vi "Sprite.vi"(5 "Pause":bool, 7 "Skip":bool, 8 "error in (no error)":errorcluster, 9 "Skip to Frame":i32=1 min=1, 10 "Sprite Sequence":T1, 11 "Sprite Name":string) -> (0 "error out":errorcluster, 1 "Next Fame":i32, 2 "Frame Output":picture, 3 "Sprite Name Out":string)   [LabVIEW 2020]
uses:
  Stickman State.ctl
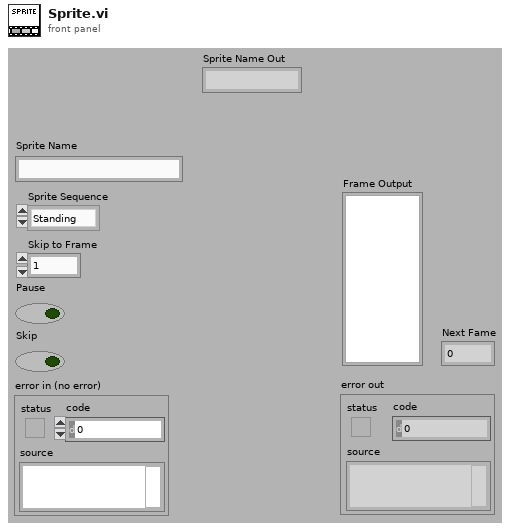
[diagram p1: front panel]
types:
  T1 = typedef "Stickman State.ctl" = enum16{"Standing", "Walking"}
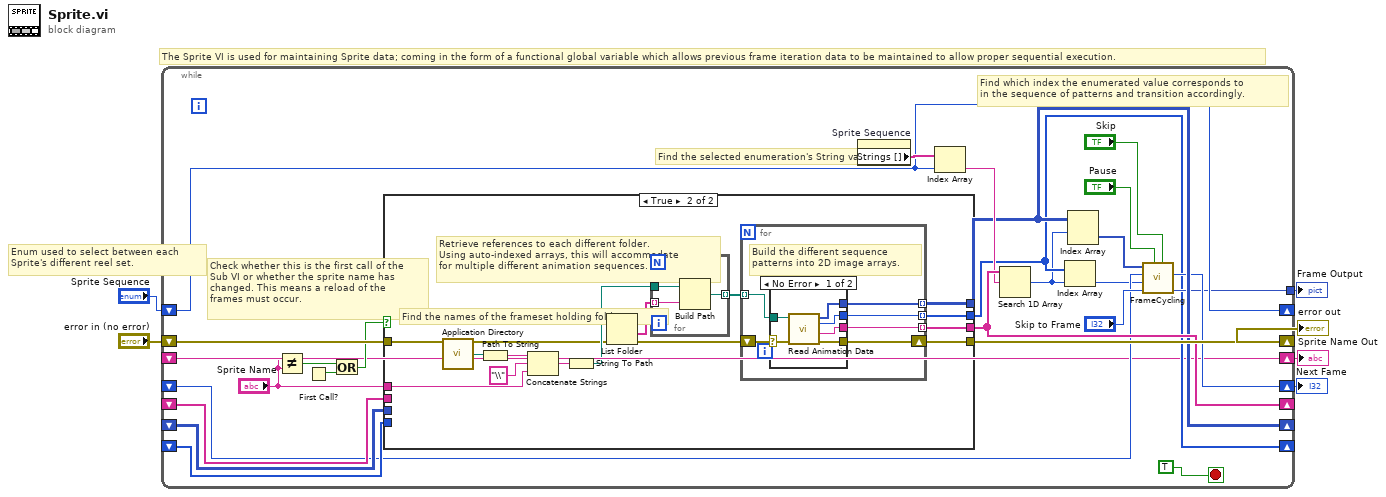
[diagram p0: block diagram]
diagram:
  # "Enum used to select between each\nSprite's different reel set."
  # "The Sprite VI is used for maintaining Sprite data; coming in the form of a functional global variable which allows previous frame iteration data to be maintained to allow proper sequential execution."
  n1 = while {
    shift-right: [w17] -> w2
    shift-left: _ -> [w18]
    shift-right: [w26] -> _
    shift-left: "Sprite Sequence" -> [w26]
    shift-right: [w23] -> _
    shift-left: _ -> [w31]
    shift-right: [w30] -> w4
    shift-left: "error in (no error)" -> [w32]
    shift-right: [w14] -> _
    shift-left: _ -> [w29]
    shift-right: [w25] -> _
    shift-left: _ -> [w28]
    tunnel: [w16] -> w3
    shift-right: ["Sprite Name"] -> w1
    shift-left: _ -> [w8]
    stop <- TRUE stop-if-true
    # "Find which index the enumerated value corresponds to\nin the sequence of patterns and transition accordingly."
    # "Find the selected enumeration's String value."
    # "Check whether this is the first call of the\nSub VI or whether the sprite name has\nchanged. This means a reload of the\nframes must occur."
    n2 = Not Equal?(x=w8, y="Sprite Name") -> (x != y?=w11:bool)
    n3 = First Call?() -> (First Call?: T/F=w10:bool)
    n4 = Or(x=w11, y=w10) -> (x .or. y?=w9:bool)
    n5 = case shown="True" w9 {
      tunnel: [w35 w50] -> w23
      tunnel: w32 -> [w36 w41]
      tunnel: w31 -> [w35 _]
      tunnel: [w36 w49] -> w30
      tunnel: [w34 w48] -> w14
      tunnel: [w33 w47] -> w25
      tunnel: w29 -> [w34 _]
      tunnel: w28 -> [w33 _]
      tunnel: "Sprite Name" -> [_ w38]
      frame False {
      }
      frame True {
        # "Retrieve references to each different folder.\nUsing auto-indexed arrays, this will accommodate\nfor multiple different animation sequences."
        # "Find the names of the frameset holding folders."
        n6 = call <vilib>:"Application Directory.vi"() -> ("Application Directory"=w37:path)
        n7 = Path To String(path=w37) -> (string=w46:string)
        n8 = Concatenate Strings(w46, "\\" ("string"), w38) -> (w45:string)
        n9 = String To Path(string=w45) -> (path=w43:path)
        n10 = List Folder(path=w43, error in=w41) -> (folder names=w44:string[], error out=w40:errorcluster)  [unwired: 2 in, 2 out]
        n11 = for {
          tunnel: w44 -> [w52] mode=indexing
          tunnel: w43 -> [w53]
          tunnel: [w51] -> w39 mode=indexing
          n12 = Build Path(base path=w53, name or relative path=w52) -> (appended path=w51:path)
        }
        n13 = for {
          tunnel: w39 -> [w59] mode=indexing
          tunnel: [w56] -> w50 mode=indexing
          shift-right: [w58] -> w49
          shift-left: w40 -> [w57]
          tunnel: [w55] -> w48 mode=indexing
          tunnel: [w54] -> w47 mode=indexing
          # "Build the different sequence\npatterns into 2D image arrays."
          n14 = case shown="No Error" w57 {
            selector: w57 -> [w65 w66]
            tunnel: w59 -> [w64 _]
            tunnel: [w63 _] -> w56
            tunnel: [w62 w66] -> w58
            tunnel: [w61 _] -> w55
            tunnel: [w60 _] -> w54
            frame No Error {
              n15 = call "Read Animation Data.vi"("error in (no error)"=w65, "Animation Path"=w64) -> ("error out"=w62:errorcluster, "Animation Set Name"=w60:string, "Total Number of Frames"=w61:i32, "Animation Reel"=w63:picture[])  [unwired: 6 in]
            }
            frame Error {
            }
          }
        }
      }
    }
    n16 = property on="Sprite Sequence" class="Enum (strict)"() -> ("Strings []"=w27:string[])  [unwired: 2 in, 2 out]
    n17 = Index Array(array=w27, index=w26) -> (element=w24:string)
    n18 = Search 1D Array(1D array=w25, element=w24) -> (index of element=w13:i32)  [unwired: 1 in]
    n19 = Index Array(array=w14, index=w13) -> (element=w12:i32)
    n20 = Index Array(array=w23, index (row)=w13) -> (element=w15:picture[])  [unwired: 1 in]
    n21 = call "FrameCycling.vi"("Skip"="Skip", "Pause"="Pause", "Skip to Frame"="Skip to Frame", "Total Reel Frames"=w12, "Current Frame"=w18, "Animation Reel In"=w15) -> ("Frame Output"=w16:picture, "Next Fame"=w17:i32)  [unwired: 3 in, 1 out]
  }
  "error out" <- w4
  "Frame Output" <- w3
  "Next Fame" <- w2
  "Sprite Name Out" <- w1
